vi "Configure DC Bias Voltage.vi"(0 "VISA resource name":refnum<visa-resource-name>, 1 "DC Bias":bool caption="BIAS", 2 "DC Bias Voltage (0)":dbl min=-2.5 max=2.5 step=0.01, 3 "error in (no error)":errorcluster) -> (7 "VISA resource name out":refnum<visa-resource-name>, 10 "error out":errorcluster)   [LabVIEW 2021, in "LCR Meter.lvlib"]
doc: "Sets the DC BIAS switch to ON or OFF, and sets the DC bias voltage value."
uses:
  LCR Meter.lvlib
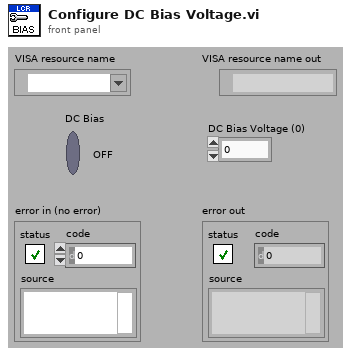
[diagram p1: front panel]
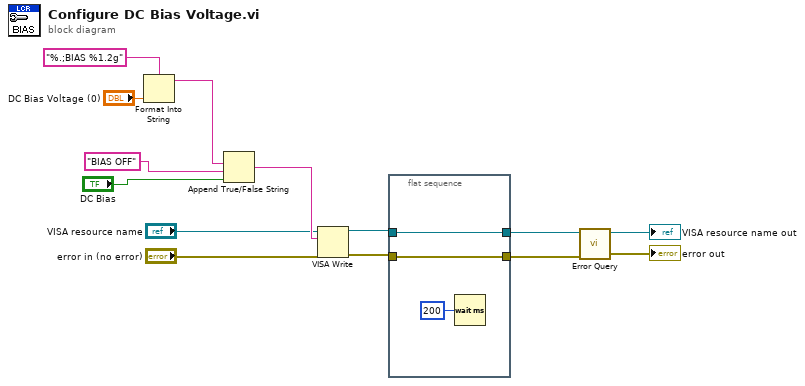
[diagram p0: block diagram]
diagram:
  n1 = Format Into String(format string="%.;BIAS %1.2g", "DC Bias Voltage (0)") -> (resulting string=w9:string)  [unwired: 2 in, 1 out]
  n2 = Append True/False String(1:"DC Bias", 2:"BIAS OFF", 3:w9) -> (0:w7:string)  [unwired: 1 in]
  n3 = VISA Write(VISA resource name="VISA resource name", write buffer=w7, error in (no error)="error in (no error)") -> (VISA resource name out=w4:refnum<visa-resource-name>, error out=w3:errorcluster)  [unwired: 1 out]
  n4 = flat-sequence {
    tunnel: [w17] -> w2
    tunnel: w4 -> [w17]
    tunnel: w3 -> [w16]
    tunnel: [w16] -> w1
    frame #0 {
      n5 = Wait (ms)(milliseconds to wait=u32 200) -> ()  [unwired: 1 out]
    }
  }
  n6 = call "Error Query.vi"("error in (no error)"=w1, "VISA resource name"=w2) -> ("error out"=→"error out":errorcluster, "VISA resource name out"=→"VISA resource name out":refnum<visa-resource-name>)  [unwired: 6 in, 2 out]
